vi "subCloseSubDlg.vi"(0 "subDlgRefs":refnum<vi>[](array[refnum]), 1 "Reference":T1, 2 "OK Pressed":bool) -> ()   [LabVIEW 2020]
uses:
  <vilib>/express/express shared/propPageData.ctl
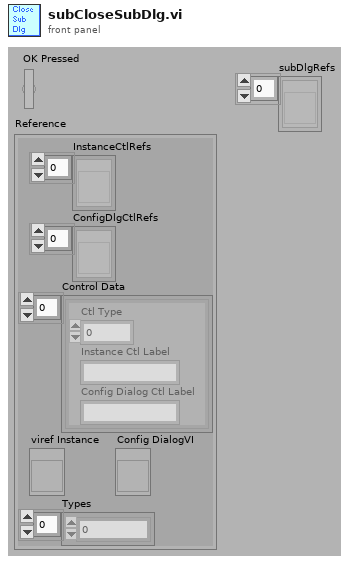
[diagram p1: front panel]
types:
  T1 = typedef "propPageData.ctl" = cluster{"InstanceCtlRefs":refnum<vi>[], "ConfigDlgCtlRefs":refnum<vi>[], "Control Data":cluster{"Ctl Type":u16, "Instance Ctl Label":string, "Config Dialog Ctl Label":string}[], "viref Instance":refnum<vi>, "Types":i32[], "Config DialogVI":refnum<vi>}
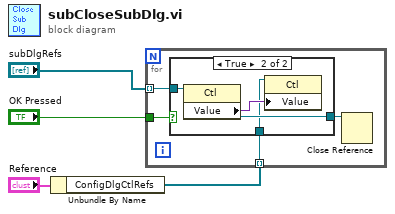
[diagram p0: block diagram]
diagram:
  n1 = Unbundle By Name("Reference") -> ("ConfigDlgCtlRefs"=w1:refnum<vi>[])
  n2 = for {
    tunnel: "OK Pressed" -> [w7]
    tunnel: "subDlgRefs" -> [w6] mode=indexing
    tunnel: w1 -> [w5] mode=indexing
    n3 = case shown="True" w7 {
      tunnel: [w9 w12] -> w8
      tunnel: w6 -> [w9 w11]
      tunnel: w5 -> [_ w10]
      frame False {
      }
      frame True {
        n4 = property class="Ctl"(reference=w11) -> (reference out=w12:refnum<vi>, "Value"=w13:variant)  [unwired: 1 in, 1 out]
        n5 = property class="Ctl"(reference=w10, "Value"=w13) -> ()  [unwired: 1 in, 2 out]
      }
    }
    n6 = Close Reference(reference=w8) -> ()  [unwired: 1 in, 1 out]
  }
